vi "Start Sync.vi"(8 "error in (no error)":errorcluster, 11 "gRPC Server in":refnum<class "RouteGuide.lvclass">) -> (0 "error out":errorcluster, 3 "gRPC Server out":refnum<class "RouteGuide.lvclass">)   [LabVIEW 2019, in "Generated_server.lvlib" / "RouteGuide.lvclass"]
uses:
  RouteGuide.lvclass
  RPC Messages/routeguide_Feature.ctl
  RPC Messages/routeguide_Point.ctl
  RPC Messages/routeguide_RouteSummary.ctl
  RouteGuide.lvclass/RouteGuide.ctl
  <vilib>/gRPC/LabVIEW gRPC Library/grpc-lvsupport-release.lvlib
  Generated_server.lvlib
panel:
  in  "?":T1
  in  "?":T2
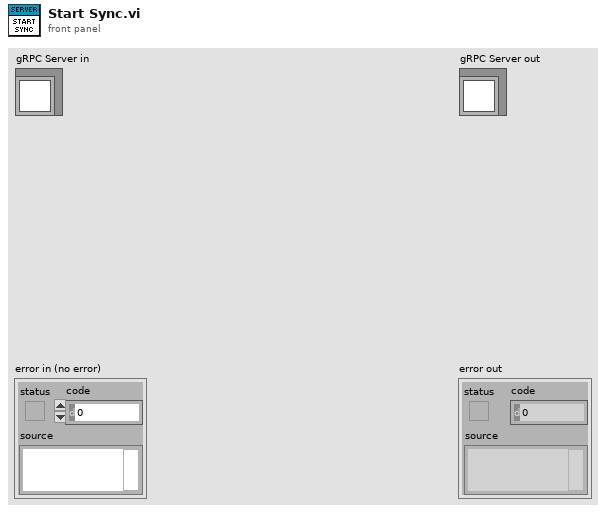
[diagram p1: front panel]
types:
  T1 = typedef "Generated_server.lvlib/routeguide_RouteSummary.ctl" = cluster{"point_count":i32, "feature_count":i32, "distance":i32, "elapsed_time":i32}
  T2 = typedef "Generated_server.lvlib/routeguide_Feature.ctl" = cluster{"name":string, "location":T3}
  T3 = typedef "Generated_server.lvlib/routeguide_Point.ctl" = cluster{"latitude":i32, "longitude":i32}
  T4 = typedef "Generated_server.lvlib/RouteGuide.lvclass/Server Internal UEs.ctl" = cluster{"RouteGuide GetFeature Internal UE":refnum<user-event>, "RouteGuide ListFeatures Internal UE":refnum<user-event>, "RouteGuide RecordRoute Internal UE":refnum<user-event>, "RouteGuide RouteChat Internal UE":refnum<user-event>}
  T5 = typedef "Generated_server.lvlib/RouteGuide.lvclass/Server gRPC UEs.ctl" = cluster{"RouteGuide GetFeature gRPC UE":refnum<user-event>, "RouteGuide ListFeatures gRPC UE":refnum<user-event>, "RouteGuide RecordRoute gRPC UE":refnum<user-event>, "RouteGuide RouteChat gRPC UE":refnum<user-event>}
  T6 = typedef "grpc-lvsupport-release.lvlib/grpcId.ctl" = u64
  T7 = typedef "Generated_server.lvlib/routeguide_Rectangle.ctl" = cluster{"lo":T3, "hi":T3}
  T8 = typedef "Generated_server.lvlib/routeguide_RouteNote.ctl" = cluster{"location":T3, "message":string}
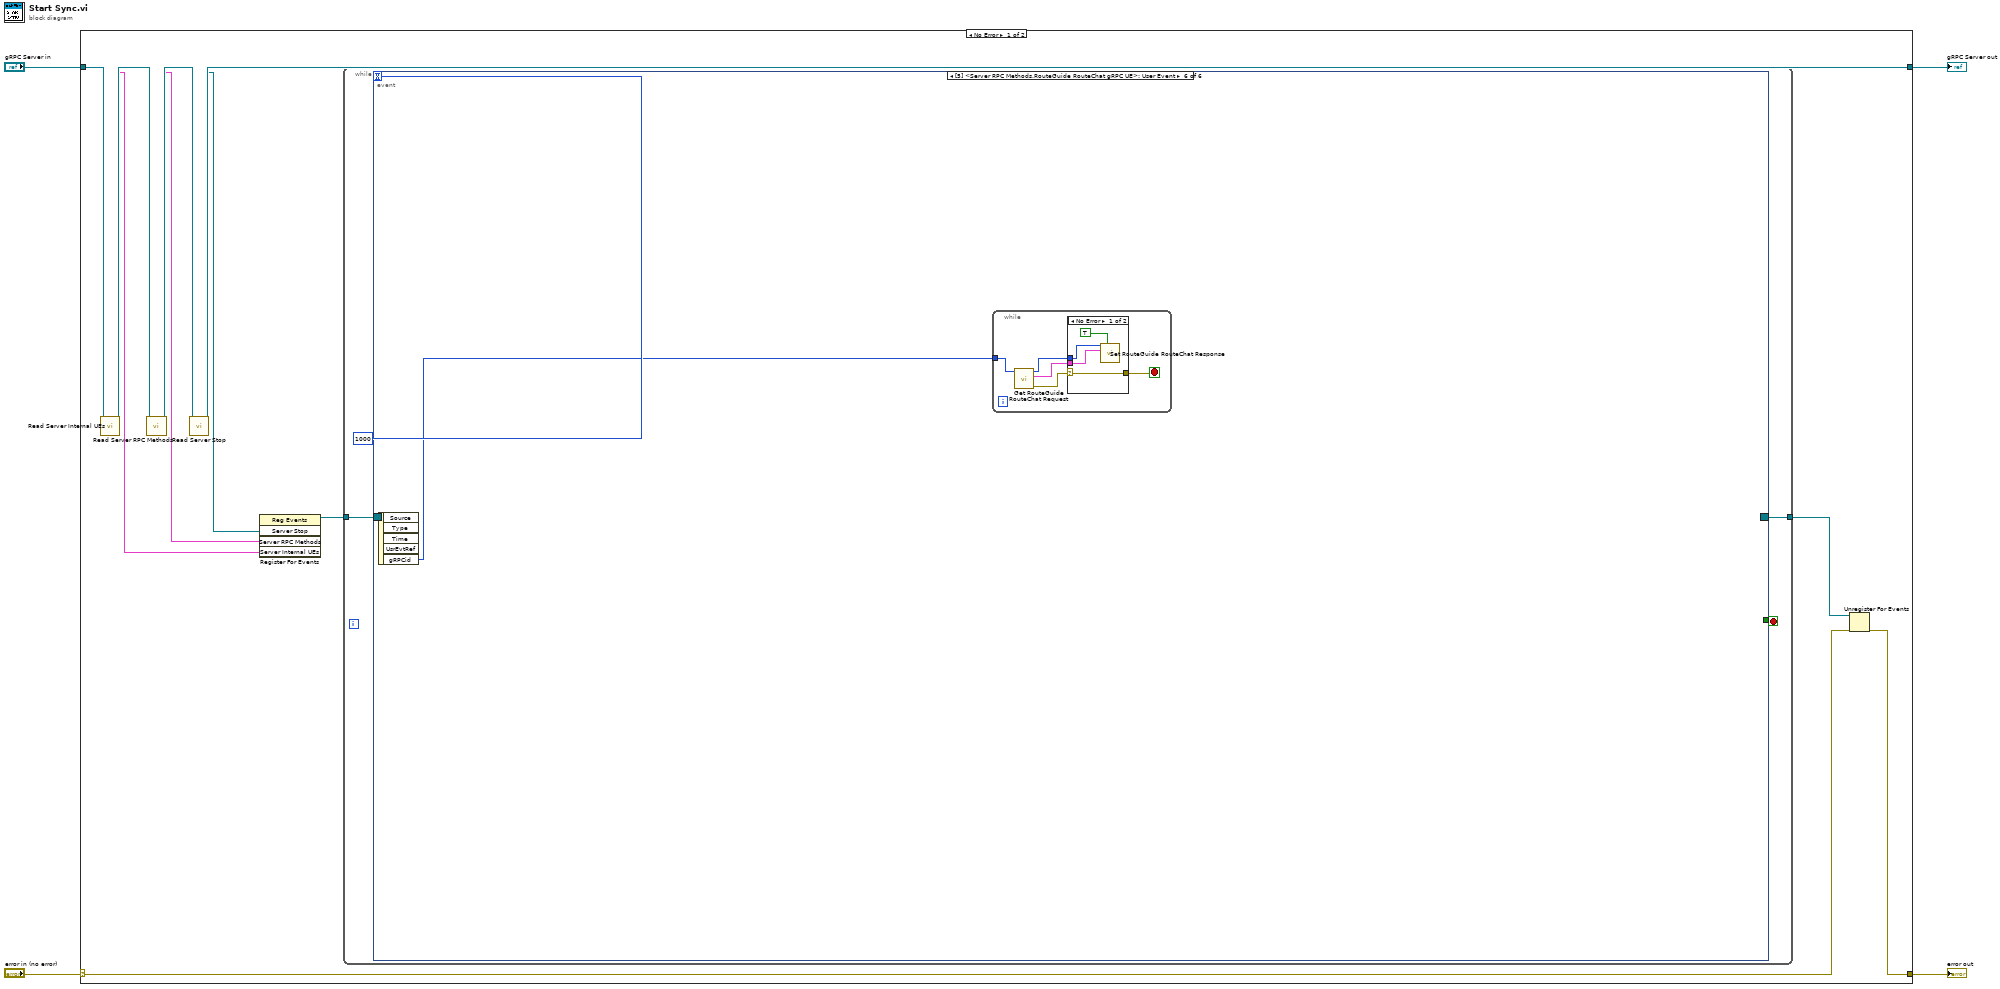
[diagram p0: block diagram]
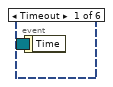
[diagram p2: hidden frame]
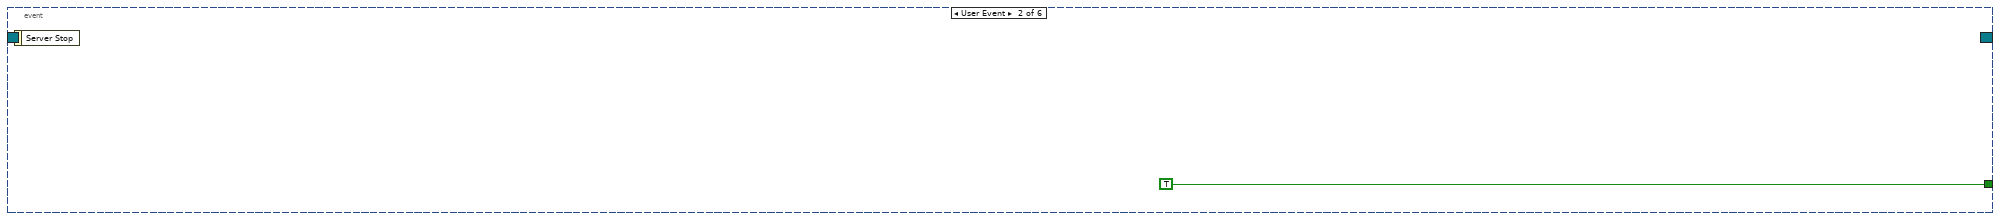
[diagram p3: hidden frame]
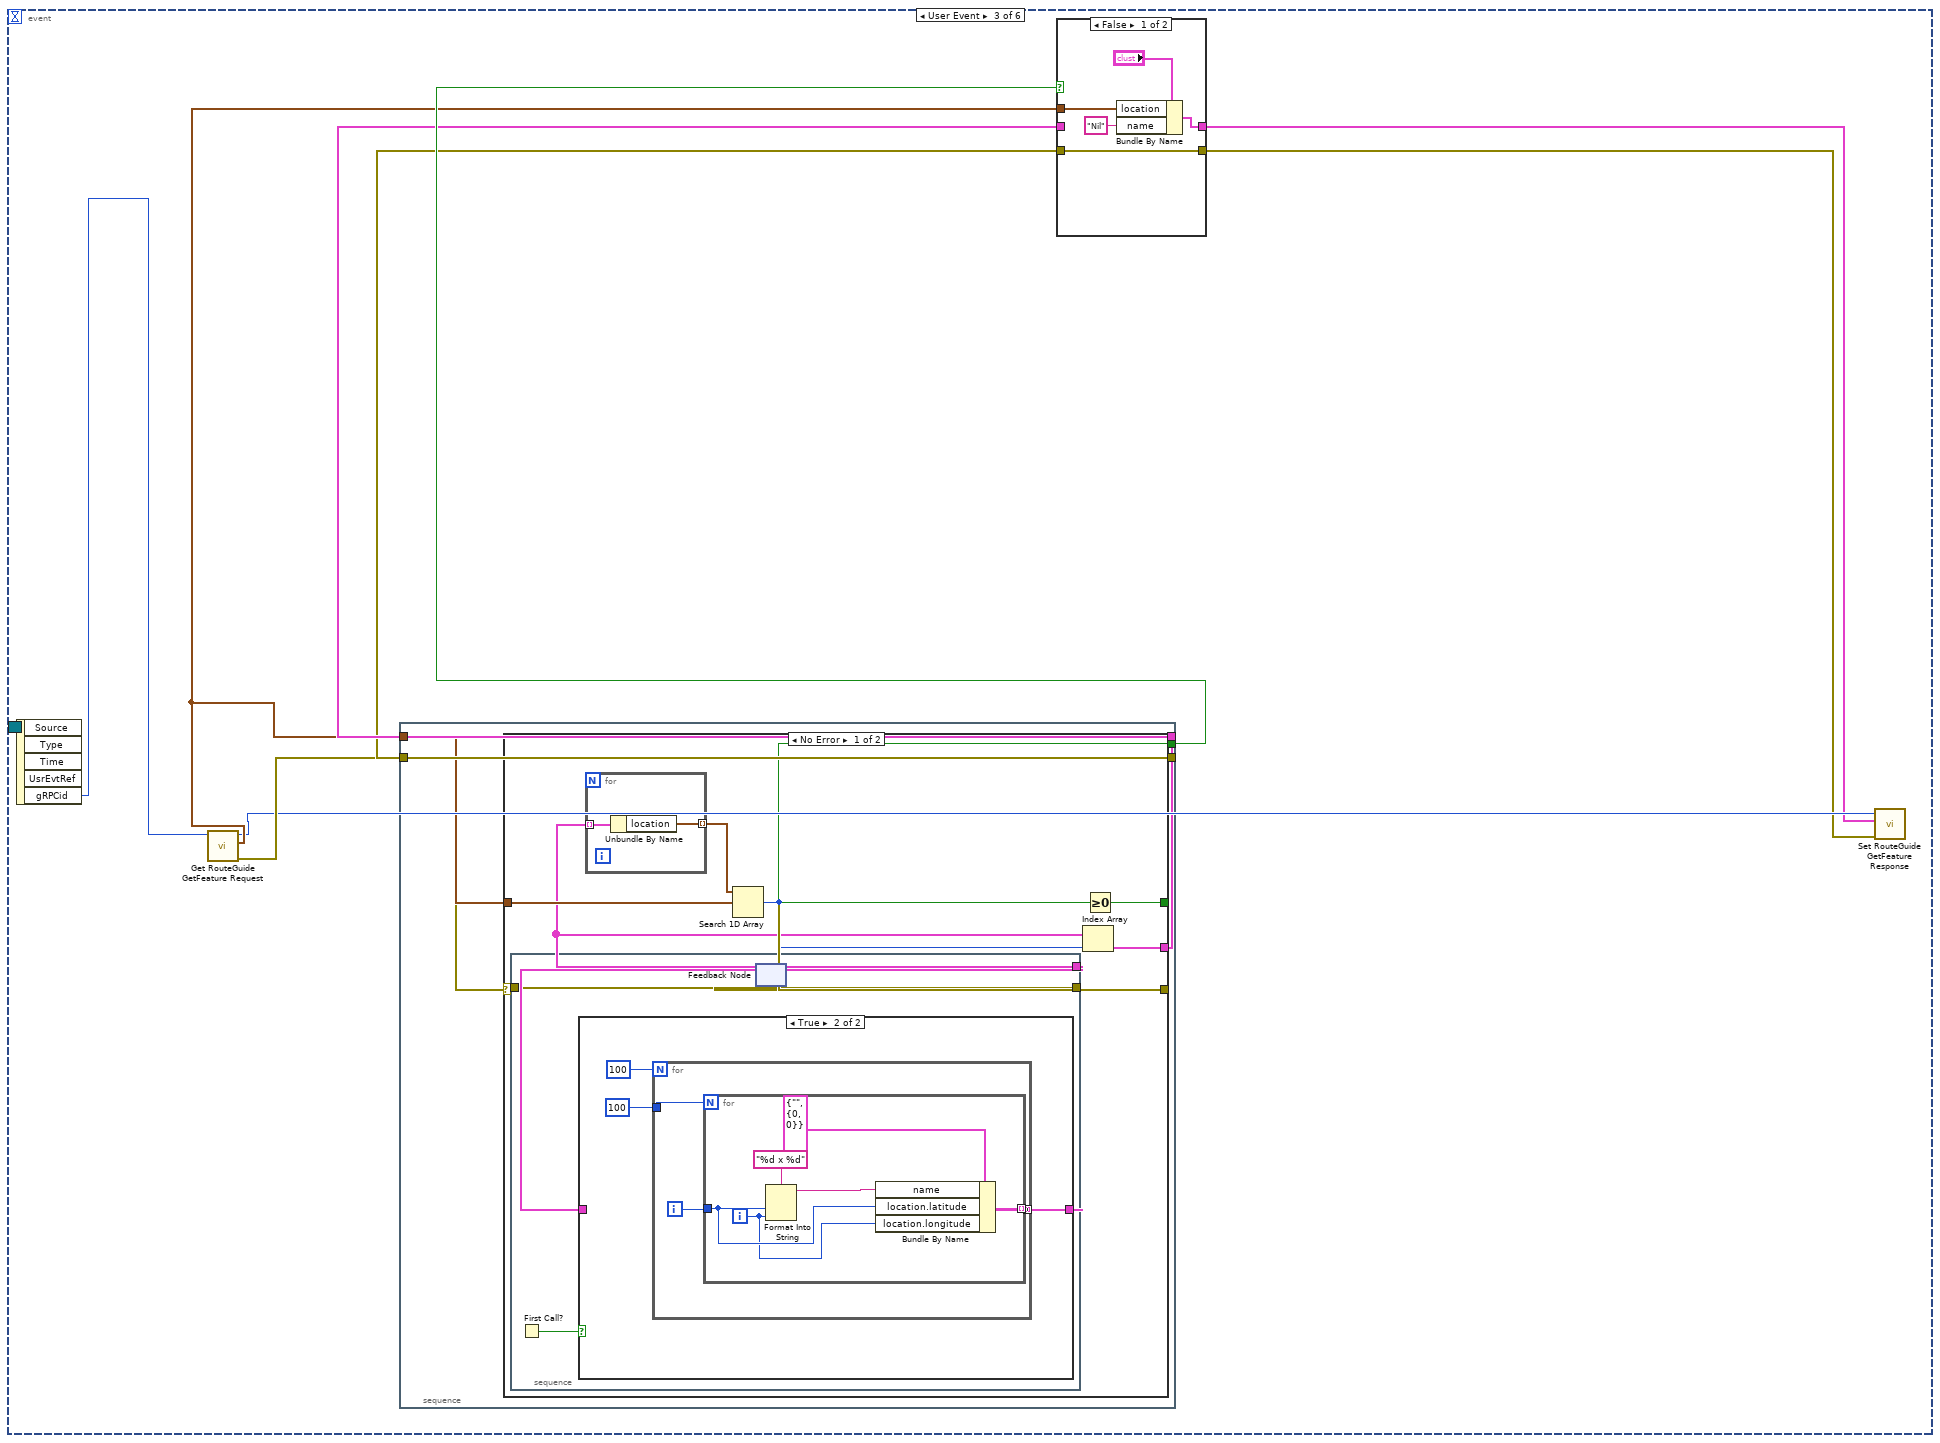
[diagram p4: hidden frame]
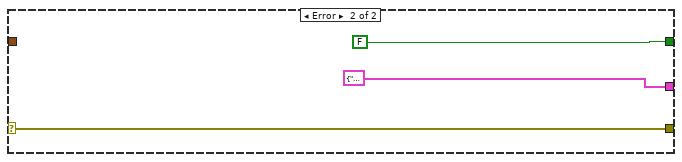
[diagram p6: hidden frame]
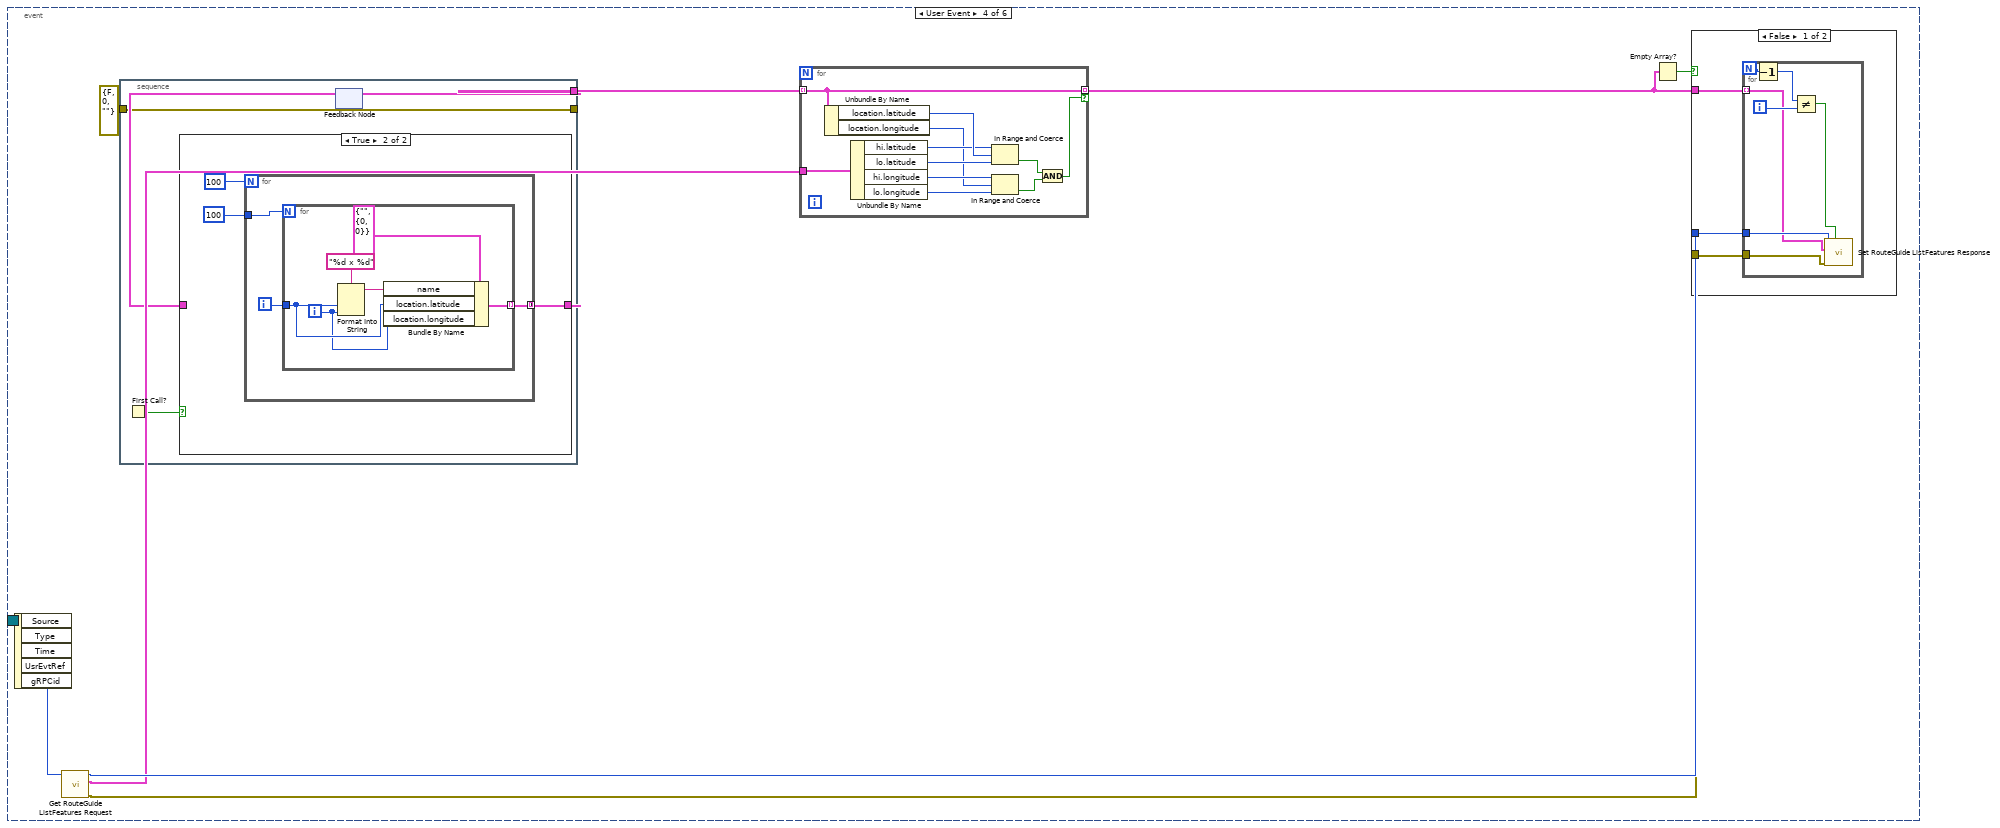
[diagram p8: hidden frame]
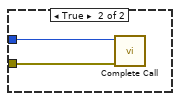
[diagram p10: hidden frame]
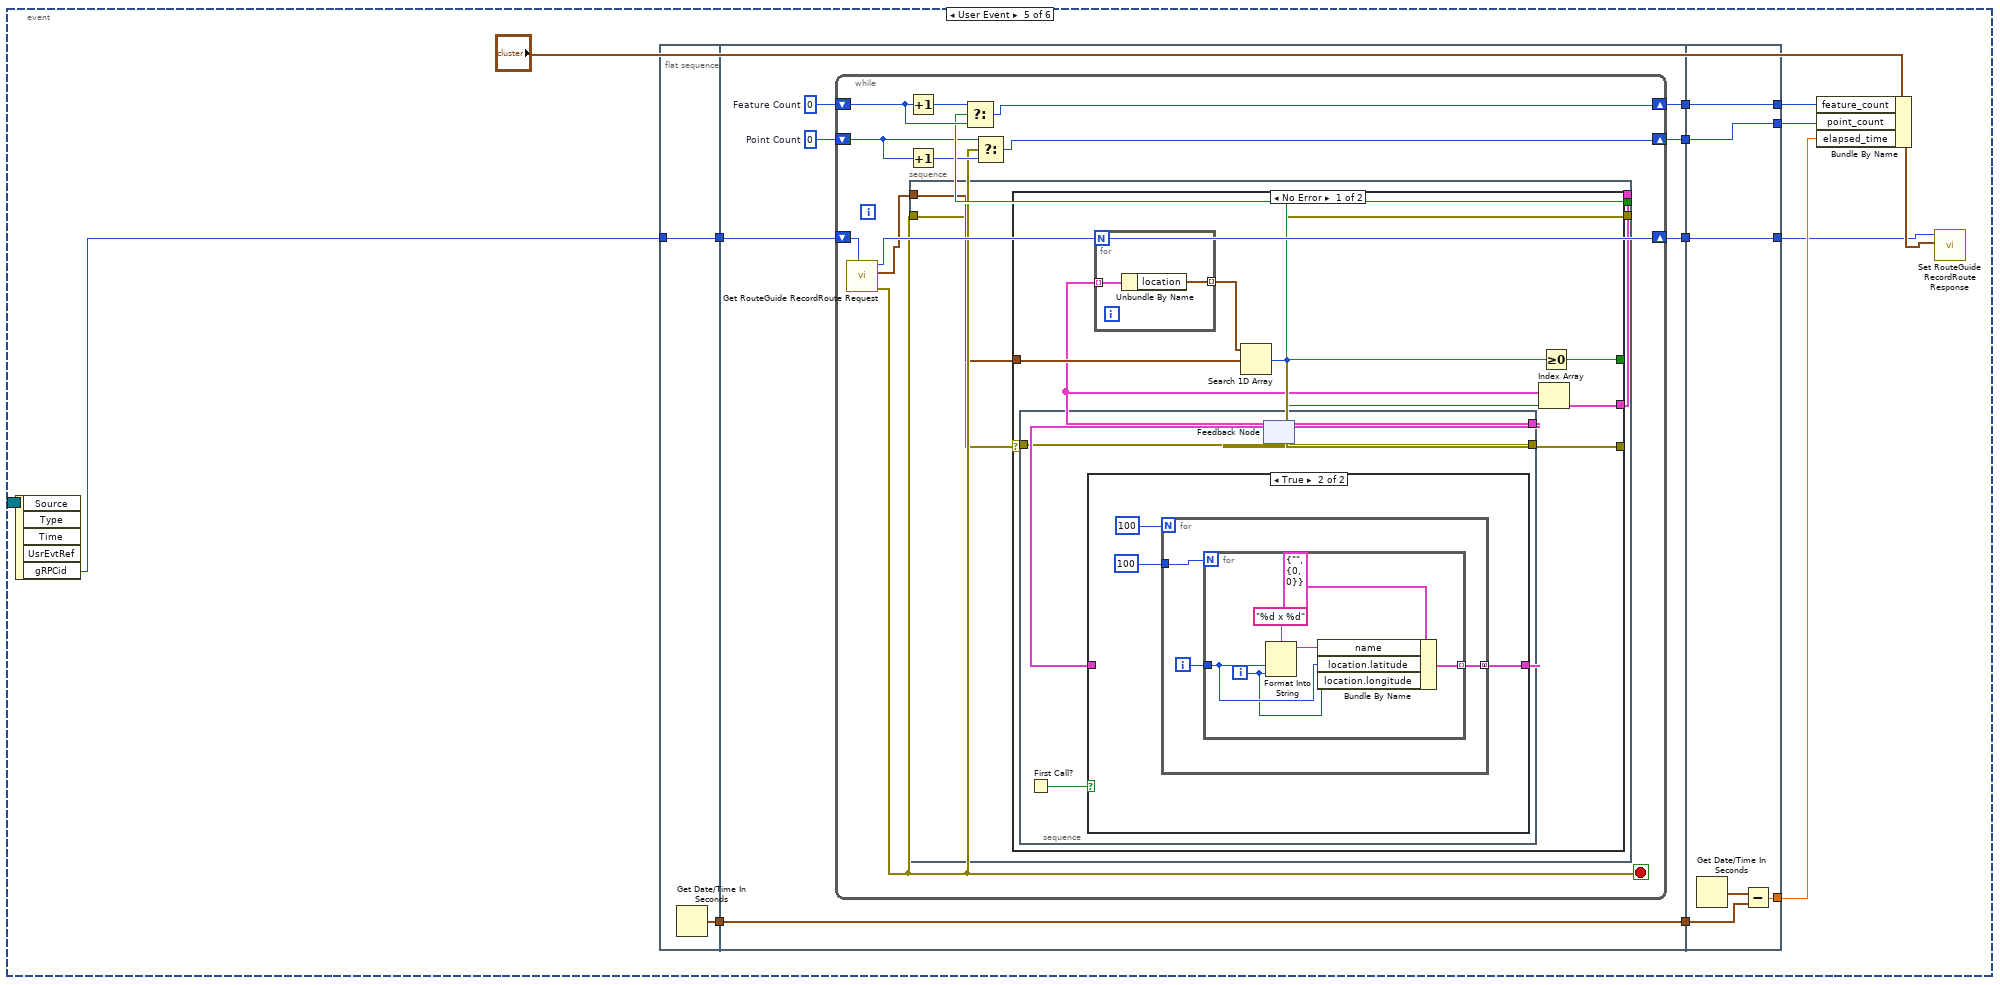
[diagram p11: hidden frame]
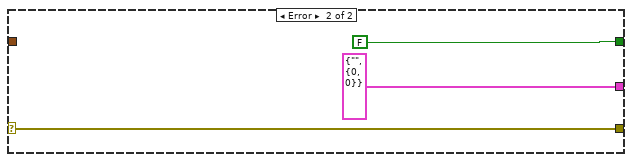
[diagram p13: hidden frame]
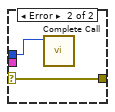
[diagram p14: hidden frame]
diagram:
  n1 = case shown="No Error" "error in (no error)" {
    selector: "error in (no error)" -> [w9 w207]
    tunnel: [w8 w207] -> w3
    tunnel: [w6 w206] -> w1
    tunnel: "gRPC Server in" -> [w15 w206]
    frame No Error {
      n2 = call "Read Server Internal UEs.vi"("SignalGeneratorService in"=w15) -> ("Server Internal UEs"=w13:T4, "SignalGeneratorService out"=w14:refnum<class "RouteGuide.lvclass">)  [unwired: 8 in, 1 out]
      n3 = call "Read Server RPC Methods.vi"("SignalGeneratorService in"=w14) -> ("Server RPC Methods"=w7:T5, "SignalGeneratorService out"=w12:refnum<class "RouteGuide.lvclass">)  [unwired: 8 in, 1 out]
      n4 = call-dynamic "Read Server Stop.vi"("iService in"=w12) -> ("Server Stop"=w5:refnum<user-event>, "iService out"=w6:refnum<class "RouteGuide.lvclass">)  [unwired: 8 in, 1 out]
      n5 = register-events(w5, w7, w13) -> (reference out=w11:refnum<event-registration>)  [unwired: 2 in, 1 out]
      n6 = while {
        tunnel: w11 -> [w19]
        tunnel: [w17] -> w10
        stop <- w18 stop-if-true
        n7 = event "RPC Methods Event Structure" shown="[5] <Server RPC Methods.RouteGuide RouteChat gRPC UE>: User Event" {
          selector: w19 -> [_ _ _ _ _ _]
          dyn-events: [_ _ _ _ _ _] -> w17
          timeout: 1000 -> [_ _ _ _ _ _]
          tunnel: [_ TRUE _ _ _ _] -> w18
          event Timeout {
            n8 = event-data() -> ()  [unwired: 1 in, 1 out]
          }
          event User Event {
            n9 = event-data() -> ()  [unwired: 1 in, 1 out]
          }
          event User Event {
            n10 = event-data() -> ("gRPCid"=w24:T6)  [unwired: 1 in, 4 out]
            n11 = call "Get RouteGuide GetFeature Request.vi"("gRPCid"=w24) -> ("error out"=w26:errorcluster, "Message Data"=w25:T3, "gRPCid out"=w23:T6)  [unwired: 8 in]
            n12 = stacked-sequence {
              tunnel: [w31] -> w27
              tunnel: [w34] -> w29
              tunnel: [w33] -> w28
              tunnel: w26 -> [w30]
              tunnel: w25 -> [w32]
              frame #0 {
                n13 = case shown="No Error" w30 {
                  selector: w30 -> [w42 w64]
                  tunnel: [w41 w64] -> w31
                  tunnel: w32 -> [w39 _]
                  tunnel: [w36 cluster{"name":string, "routeguide_Point":T3} {"name"="", "routeguide_Point"={"latitude"=0, "longitude"=0}} ("routeguide_Feature")] -> w33
                  tunnel: [w35 FALSE] -> w34
                  frame No Error {
                    n14 = stacked-sequence {
                      tunnel: [w43] -> w41
                      tunnel: [w45] -> w38
                      tunnel: w42 -> [w43]
                      frame #0 {
                        n15 = First Call?() -> (First Call?: T/F=w44:bool)
                        n16 = feedback #1() -> (w46:cluster{"name":string, "location":T3}[])  [unwired: 1 in]
                        n17 = case shown="True" w44 {
                          tunnel: [w47 w48] -> w45
                          tunnel: w46 -> [w47 _]
                          frame False {
                          }
                          frame True {
                            n18 = for {
                              N: 100 -> [_]
                              tunnel: [w51] -> w48 mode=concatenating
                              tunnel: 100 -> [w53]
                              i -> [w52]
                              n19 = for {
                                N: w53 -> [_]
                                tunnel: w52 -> [w56]
                                tunnel: [w54] -> w51 mode=indexing
                                i -> [w55]
                                n20 = Format Into String(format string="%d x %d", w56, w55) -> (resulting string=w57:string)  [unwired: 2 in, 1 out]
                                n21 = Bundle By Name(cluster=cluster{"name":string, "location":T3} {"name"="", "location"={"latitude"=0, "longitude"=0}} ("routeguide_Feature"), "name"=w57, "location.latitude"=w56, "location.longitude"=w55) -> (w54:cluster{"name":string, "location":T3})
                              }
                            }
                          }
                        }
                        n22 = feedback-in #1(w45) -> ()
                      }
                    }
                    n23 = for {
                      tunnel: w38 -> [w61] mode=indexing
                      tunnel: [w60] -> w40 mode=indexing
                      n24 = Unbundle By Name(w61) -> ("location"=w60:T3)
                    }
                    n25 = Search 1D Array(1D array=w40, element=w39) -> (index of element=w37:i32)  [unwired: 1 in]
                    n26 = Index Array(array=w38, index=w37) -> (element=w36:cluster{"name":string, "location":T3})
                    n27 = Greater Or Equal To 0?(x=w37) -> (x >= 0?=w35:bool)
                  }
                  frame Error {
                  }
                }
              }
            }
            n28 = case shown="False" w29 {
              tunnel: w28 -> [_ w71]
              tunnel: w27 -> [w69 w70]
              tunnel: [w68 w71] -> w22
              tunnel: [w69 w70] -> w21
              tunnel: w25 -> [w67 _]
              frame False {
                n29 = Bundle By Name(cluster="?", "location"=w67, "name"="Nil") -> (w68:T2)
              }
              frame True {
              }
            }
            n30 = call "Set RouteGuide GetFeature Response.vi"("error in (no error)"=w21, "Message Data"=w22, "gRPCid in"=w23) -> ()  [unwired: 8 in, 1 out]
          }
          event User Event {
            n31 = event-data() -> ("gRPCid"=w72:T6)  [unwired: 1 in, 4 out]
            n32 = call "Get RouteGuide ListFeatures Request.vi"("gRPCid"=w72) -> ("error out"=w73:errorcluster, "Message Data"=w74:T7, "gRPCid out"=w75:T6)  [unwired: 8 in]
            n33 = stacked-sequence {
              tunnel: [w80] -> _
              tunnel: [w82] -> w79
              tunnel: errorcluster {"status"=FALSE, "code"=0, "source"=""} ("error in") -> [w80]
              frame #0 {
                n34 = First Call?() -> (First Call?: T/F=w81:bool)
                n35 = feedback #2() -> (w83:cluster{"name":string, "location":T3}[])  [unwired: 1 in]
                n36 = case shown="True" w81 {
                  tunnel: [w84 w86] -> w82
                  tunnel: w83 -> [w84 _]
                  frame False {
                  }
                  frame True {
                    n37 = for {
                      N: 100 -> [_]
                      tunnel: [w89] -> w86 mode=concatenating
                      tunnel: 100 -> [w88]
                      i -> [w90]
                      n38 = for {
                        N: w88 -> [_]
                        tunnel: w90 -> [w93]
                        tunnel: [w91] -> w89 mode=indexing
                        i -> [w92]
                        n39 = Format Into String(format string="%d x %d", w93, w92) -> (resulting string=w94:string)  [unwired: 2 in, 1 out]
                        n40 = Bundle By Name(cluster=cluster{"name":string, "location":T3} {"name"="", "location"={"latitude"=0, "longitude"=0}} ("routeguide_Feature"), "name"=w94, "location.latitude"=w93, "location.longitude"=w92) -> (w91:cluster{"name":string, "location":T3})
                      }
                    }
                  }
                }
                n41 = feedback-in #2(w82) -> ()
              }
            }
            n42 = for {
              tunnel: w79 -> [w110] mode=indexing
              tunnel: w74 -> [w119]
              tunnel: [w110] -> w77 mode=indexing if=w109
              n43 = Unbundle By Name(w110) -> ("location.latitude"=w118:i32, "location.longitude"=w113:i32)
              n44 = Unbundle By Name(w119) -> ("hi.latitude"=w117:i32, "lo.latitude"=w116:i32, "hi.longitude"=w115:i32, "lo.longitude"=w114:i32)
              n45 = In Range and Coerce(upper limit=w117, x=w118, lower limit=w116) -> (In Range?=w111:bool)  [unwired: 1 out]
              n46 = In Range and Coerce(upper limit=w115, x=w113, lower limit=w114) -> (In Range?=w112:bool)  [unwired: 1 out]
              n47 = And(x=w111, y=w112) -> (x .and. y?=w109:bool)
            }
            n48 = Empty Array?(array=w77) -> (empty?=w78:bool)
            n49 = case shown="False" w78 {
              tunnel: w75 -> [w99 w107]
              tunnel: w73 -> [w98 w108]
              tunnel: w77 -> [w97 _]
              frame False {
                n50 = for {
                  N -> [w106]
                  tunnel: w99 -> [w102]
                  tunnel: w98 -> [w100]
                  tunnel: w97 -> [w101] mode=indexing
                  i -> [w105]
                  n51 = Decrement(x=w106) -> (x-1=w104:i32)
                  n52 = Not Equal?(x=w104, y=w105) -> (x != y?=w103:bool)
                  n53 = call "Set RouteGuide ListFeatures Response.vi"("Streaming? (F)"=w103, "error in (no error)"=w100, "Message Data"=w101, "gRPCid in"=w102) -> ()  [unwired: 7 in, 1 out]
                }
              }
              frame True {
                n54 = call <vilib>:"Complete Call.vi"("gRPCid"=w107, "error in"=w108) -> ()  [unwired: 8 in, 1 out]
              }
            }
          }
          event User Event {
            n55 = event-data() -> ("gRPCid"=w123:T6)  [unwired: 1 in, 4 out]
            n56 = flat-sequence {
              tunnel: w123 -> [w134]
              tunnel: [w134] -> w132
              tunnel: [w133] -> w131
              tunnel: w132 -> [w141]
              tunnel: [w140] -> w130
              tunnel: [w135] -> w129
              tunnel: [w138] -> w128
              tunnel: w131 -> [w137]
              tunnel: [w137] -> w127
              tunnel: [w192] -> w126
              tunnel: [w193] -> w120
              tunnel: w130 -> [w193]
              tunnel: w129 -> [w192]
              tunnel: [w191] -> w125
              tunnel: w128 -> [w191]
              tunnel: w127 -> [w189]
              tunnel: [w188] -> w124
              frame #0 {
                n57 = Get Date/Time In Seconds() -> (seconds since 1Jan1904=w133:timestamp)
              }
              frame #1 {
                w136 = 0  # Point Count
                w139 = 0  # Feature Count
                n58 = while {
                  shift-right: [w144] -> w140
                  shift-left: w141 -> [w145]
                  shift-right: [w152] -> w138
                  shift-left: w139 -> [w151]
                  shift-right: [w148] -> w135
                  shift-left: w136 -> [w146]
                  stop <- w143 stop-if-true
                  n59 = call "Get RouteGuide RecordRoute Request.vi"("gRPCid"=w145) -> ("error out"=w143:errorcluster, "Message Data"=w142:T3, "gRPCid out"=w144:T6)  [unwired: 8 in]
                  n60 = Increment(x=w151) -> (x+1=w150:i32)
                  n61 = Increment(x=w146) -> (x+1=w147:i32)
                  n62 = stacked-sequence {
                    tunnel: [w154] -> _
                    tunnel: [w157] -> w149
                    tunnel: [w156] -> _
                    tunnel: w143 -> [w153]
                    tunnel: w142 -> [w155]
                    frame #0 {
                      n63 = case shown="No Error" w153 {
                        selector: w153 -> [w165 w187]
                        tunnel: [w164 w187] -> w154
                        tunnel: w155 -> [w162 _]
                        tunnel: [w159 cluster{"name":string, "routeguide_Point":T3} {"name"="", "routeguide_Point"={"latitude"=0, "longitude"=0}} ("routeguide_Feature")] -> w156
                        tunnel: [w158 FALSE] -> w157
                        frame No Error {
                          n64 = stacked-sequence {
                            tunnel: [w166] -> w164
                            tunnel: [w168] -> w161
                            tunnel: w165 -> [w166]
                            frame #0 {
                              n65 = First Call?() -> (First Call?: T/F=w167:bool)
                              n66 = feedback #3() -> (w169:cluster{"name":string, "location":T3}[])  [unwired: 1 in]
                              n67 = case shown="True" w167 {
                                tunnel: [w170 w172] -> w168
                                tunnel: w169 -> [w170 _]
                                frame False {
                                }
                                frame True {
                                n68 = for {
                                N: 100 -> [_]
                                tunnel: [w175] -> w172 mode=concatenating
                                tunnel: 100 -> [w174]
                                i -> [w176]
                                n69 = for {
                                N: w174 -> [_]
                                tunnel: w176 -> [w179]
                                tunnel: [w177] -> w175 mode=indexing
                                i -> [w178]
                                n70 = Format Into String(format string="%d x %d", w179, w178) -> (resulting string=w180:string)  [unwired: 2 in, 1 out]
                                n71 = Bundle By Name(cluster=cluster{"name":string, "location":T3} {"name"="", "location"={"latitude"=0, "longitude"=0}} ("routeguide_Feature"), "name"=w180, "location.latitude"=w179, "location.longitude"=w178) -> (w177:cluster{"name":string, "location":T3})
                                }
                                }
                                }
                              }
                              n72 = feedback-in #3(w168) -> ()
                            }
                          }
                          n73 = for {
                            tunnel: w161 -> [w184] mode=indexing
                            tunnel: [w183] -> w163 mode=indexing
                            n74 = Unbundle By Name(w184) -> ("location"=w183:T3)
                          }
                          n75 = Search 1D Array(1D array=w163, element=w162) -> (index of element=w160:i32)  [unwired: 1 in]
                          n76 = Index Array(array=w161, index=w160) -> (element=w159:cluster{"name":string, "location":T3})
                          n77 = Greater Or Equal To 0?(x=w160) -> (x >= 0?=w158:bool)
                        }
                        frame Error {
                        }
                      }
                    }
                  }
                  n78 = Select(t=w150, s=w149, f=w151) -> (s? t:f=w152:i32)
                  n79 = Select(t=w146, s=w143, f=w147) -> (s? t:f=w148:i32)
                }
              }
              frame #2 {
                n80 = Get Date/Time In Seconds() -> (seconds since 1Jan1904=w190:timestamp)
                n81 = Subtract(x=w190, y=w189) -> (x-y=w188:dbl)
              }
            }
            n82 = Bundle By Name(cluster="?", "feature_count"=w125, "point_count"=w126, "elapsed_time"=w124) -> (w121:T1)
            n83 = call "Set RouteGuide RecordRoute Response.vi"("Message Data"=w121, "gRPCid in"=w120) -> ()  [unwired: 9 in, 1 out]
          }
          event User Event {
            n84 = event-data() -> ("gRPCid"=w194:T6)  [unwired: 1 in, 4 out]
            n85 = while {
              tunnel: w194 -> [w195]
              stop <- w199 stop-if-true
              n86 = call "Get RouteGuide RouteChat Request.vi"("gRPCid"=w195) -> ("error out"=w196:errorcluster, "Message Data"=w197:T8, "gRPCid out"=w198:T6)  [unwired: 8 in]
              n87 = case shown="No Error" w196 {
                selector: w196 -> [w203 w205]
                tunnel: w198 -> [w202 w204]
                tunnel: w197 -> [w201 _]
                tunnel: [w203 w205] -> w199
                frame No Error {
                  n88 = call "Set RouteGuide RouteChat Response.vi"("Streaming? (F)"=TRUE ("Streeming? (F)"), "Message Data"=w201, "gRPCid in"=w202) -> ()  [unwired: 8 in, 1 out]
                }
                frame Error {
                  n89 = call <vilib>:"Complete Call.vi"("gRPCid"=w204) -> ()  [unwired: 9 in, 1 out]
                }
              }
            }
          }
        }
      }
      n90 = Unregister For Events(event registration refnum=w10, error in=w9) -> (error out=w8:errorcluster)
    }
    frame Error {
    }
  }
  "error out" <- w3
  "gRPC Server out" <- w1
